vi "Histogram by Bins.vi"(2 "Bins":T1(array[cluster]) {"upper" format="%0.2f"; "lower" format="%0.2f"}, 3 "Input Data":dbl[](array[numeric]) format="%0.2f") -> (0 "# outside":cluster{"total":i32, "above":i32, "below":i32}, 1 "Histogram":i32[](array[numeric]))   [LabVIEW 2020, in "NI_PtbyPt.lvlib"]
uses:
  <vilib>/ptbypt/NI_PtbyPt.lvlib
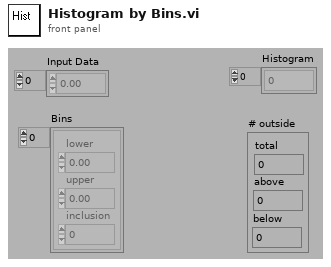
[diagram p1: front panel]
types:
  T1 = cluster{"lower":dbl, "upper":dbl, "inclusion":u32}[]
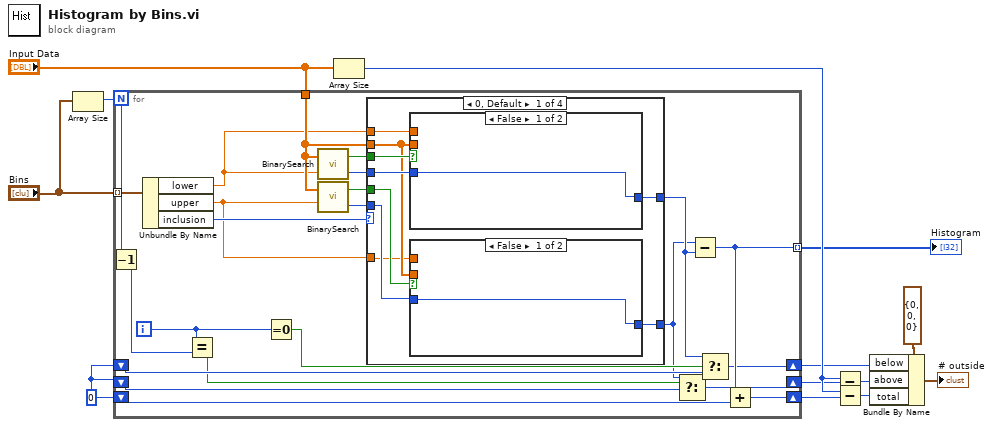
[diagram p0: block diagram]
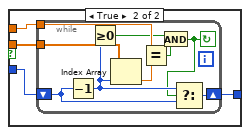
[diagram p2: hidden frame]
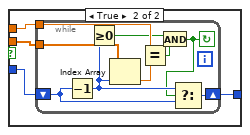
[diagram p3: hidden frame]
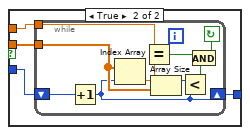
[diagram p5: hidden frame]
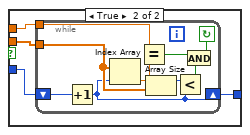
[diagram p6: hidden frame]
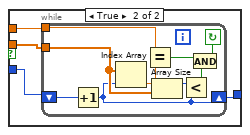
[diagram p8: hidden frame]
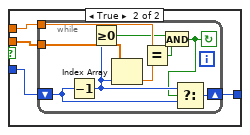
[diagram p9: hidden frame]
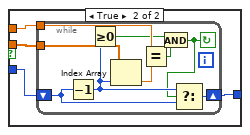
[diagram p11: hidden frame]
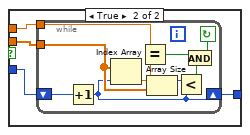
[diagram p12: hidden frame]
diagram:
  w4 = 0
  n1 = Array Size(array="Bins") -> (size(s)=w11:i32)
  n2 = for {
    N: w11 -> [w21]
    tunnel: "Bins" -> [w36] mode=indexing
    tunnel: "Input Data" -> [w31]
    tunnel: [w27] -> w3 mode=indexing
    shift-right: [w28] -> w9
    shift-left: w4 -> [w26]
    shift-right: [w23] -> w7
    shift-left: w4 -> [w24]
    shift-right: [w14] -> w5
    shift-left: w4 -> [w18]
    i -> [w22]
    n3 = Decrement(x=w21) -> (x-1=w20:i32)
    n4 = Unbundle By Name(w36) -> ("lower"=w30:dbl, "upper"=w29:dbl, "inclusion"=w35:u32)
    n5 = Equal?(x=w22, y=w20) -> (x = y?=w19:bool)
    n6 = Equal To 0?(x=w22) -> (x = 0?=w25:bool)
    n7 = call <vilib>:"BinarySearch.vi"("value searching for"=w30, "Sorted Array"=w31) -> ("index"=w17:i32, "isFound"=w32:bool)
    n8 = call <vilib>:"BinarySearch.vi"("value searching for"=w29, "Sorted Array"=w31) -> ("index"=w34:i32, "isFound"=w33:bool)
    n9 = case shown="0, Default" w35 {
      tunnel: w17 -> [w44 w81 w118 w155]
      tunnel: w34 -> [w41 w78 w115 w152]
      tunnel: w33 -> [w43 w80 w117 w154]
      tunnel: w32 -> [w45 w82 w119 w156]
      tunnel: w31 -> [w42 w79 w116 w153]
      tunnel: w30 -> [w40 w77 w114 w151]
      tunnel: w29 -> [w39 w76 w113 w150]
      tunnel: [w38 w75 w112 w149] -> w16
      tunnel: [w37 w74 w111 w148] -> w15
      frame 0, Default {
        n10 = case shown="False" w45 {
          tunnel: w44 -> [w60 w63]
          tunnel: w42 -> [_ w64]
          tunnel: w40 -> [_ w62]
          tunnel: [w60 w61] -> w38
          frame False {
          }
          frame True {
            n11 = while {
              tunnel: w62 -> [w72]
              shift-left: w63 -> [w69]
              shift-right: [w70] -> w61
              tunnel: w64 -> [w73]
              stop <- w65 continue-if-true
              n12 = Decrement(x=w69) -> (x-1=w68:i32)
              n13 = Greater Or Equal To 0?(x=w68) -> (x >= 0?=w67:bool)
              n14 = Index Array(array=w73, index=w68) -> (element=w71:dbl)
              n15 = Equal?(x=w72, y=w71) -> (x = y?=w66:bool)
              n16 = And(x=w67, y=w66) -> (x .and. y?=w65:bool)
              n17 = Select(t=w68, s=w65, f=w69) -> (s? t:f=w70:i32)
            }
          }
        }
        n18 = case shown="False" w43 {
          tunnel: w41 -> [w46 w49]
          tunnel: w42 -> [_ w48]
          tunnel: w39 -> [_ w47]
          tunnel: [w46 w50] -> w37
          frame False {
          }
          frame True {
            n19 = while {
              tunnel: w47 -> [w58]
              shift-left: w49 -> [w55]
              shift-right: [w56] -> w50
              tunnel: w48 -> [w59]
              stop <- w51 continue-if-true
              n20 = Decrement(x=w55) -> (x-1=w54:i32)
              n21 = Greater Or Equal To 0?(x=w54) -> (x >= 0?=w53:bool)
              n22 = Index Array(array=w59, index=w54) -> (element=w57:dbl)
              n23 = Equal?(x=w58, y=w57) -> (x = y?=w52:bool)
              n24 = And(x=w53, y=w52) -> (x .and. y?=w51:bool)
              n25 = Select(t=w54, s=w51, f=w55) -> (s? t:f=w56:i32)
            }
          }
        }
      }
      frame 1 {
        n26 = case shown="False" w82 {
          tunnel: w81 -> [w97 w100]
          tunnel: w79 -> [_ w101]
          tunnel: w77 -> [_ w99]
          tunnel: [w97 w98] -> w75
          frame False {
          }
          frame True {
            n27 = while {
              tunnel: w99 -> [w110]
              shift-left: w100 -> [w108]
              shift-right: [w104] -> w98
              tunnel: w101 -> [w105]
              stop <- w107 continue-if-true
              n28 = Increment(x=w108) -> (x+1=w104:i32)
              n29 = Index Array(array=w105, index=w104) -> (element=w109:dbl)
              n30 = Equal?(x=w110, y=w109) -> (x = y?=w106:bool)
              n31 = Array Size(array=w105) -> (size(s)=w103:i32)
              n32 = Less?(x=w103, y=w104) -> (x < y?=w102:bool)
              n33 = And(x=w106, y=w102) -> (x .and. y?=w107:bool)
            }
          }
        }
        n34 = case shown="False" w80 {
          tunnel: w78 -> [w83 w85]
          tunnel: w79 -> [_ w86]
          tunnel: w76 -> [_ w87]
          tunnel: [w83 w84] -> w74
          frame False {
          }
          frame True {
            n35 = while {
              tunnel: w87 -> [w96]
              shift-left: w85 -> [w94]
              shift-right: [w90] -> w84
              tunnel: w86 -> [w91]
              stop <- w93 continue-if-true
              n36 = Increment(x=w94) -> (x+1=w90:i32)
              n37 = Index Array(array=w91, index=w90) -> (element=w95:dbl)
              n38 = Equal?(x=w96, y=w95) -> (x = y?=w92:bool)
              n39 = Array Size(array=w91) -> (size(s)=w89:i32)
              n40 = Less?(x=w89, y=w90) -> (x < y?=w88:bool)
              n41 = And(x=w92, y=w88) -> (x .and. y?=w93:bool)
            }
          }
        }
      }
      frame 2 {
        n42 = case shown="False" w119 {
          tunnel: w118 -> [w134 w136]
          tunnel: w116 -> [_ w137]
          tunnel: w114 -> [_ w138]
          tunnel: [w134 w135] -> w112
          frame False {
          }
          frame True {
            n43 = while {
              tunnel: w138 -> [w146]
              shift-left: w136 -> [w143]
              shift-right: [w144] -> w135
              tunnel: w137 -> [w147]
              stop <- w139 continue-if-true
              n44 = Decrement(x=w143) -> (x-1=w142:i32)
              n45 = Greater Or Equal To 0?(x=w142) -> (x >= 0?=w141:bool)
              n46 = Index Array(array=w147, index=w142) -> (element=w145:dbl)
              n47 = Equal?(x=w146, y=w145) -> (x = y?=w140:bool)
              n48 = And(x=w141, y=w140) -> (x .and. y?=w139:bool)
              n49 = Select(t=w142, s=w139, f=w143) -> (s? t:f=w144:i32)
            }
          }
        }
        n50 = case shown="False" w117 {
          tunnel: w115 -> [w120 w122]
          tunnel: w116 -> [_ w123]
          tunnel: w113 -> [_ w124]
          tunnel: [w120 w121] -> w111
          frame False {
          }
          frame True {
            n51 = while {
              tunnel: w124 -> [w133]
              shift-left: w122 -> [w131]
              shift-right: [w127] -> w121
              tunnel: w123 -> [w128]
              stop <- w130 continue-if-true
              n52 = Increment(x=w131) -> (x+1=w127:i32)
              n53 = Index Array(array=w128, index=w127) -> (element=w132:dbl)
              n54 = Equal?(x=w133, y=w132) -> (x = y?=w129:bool)
              n55 = Array Size(array=w128) -> (size(s)=w126:i32)
              n56 = Less?(x=w126, y=w127) -> (x < y?=w125:bool)
              n57 = And(x=w129, y=w125) -> (x .and. y?=w130:bool)
            }
          }
        }
      }
      frame 3 {
        n58 = case shown="False" w156 {
          tunnel: w155 -> [w171 w173]
          tunnel: w153 -> [_ w174]
          tunnel: w151 -> [_ w175]
          tunnel: [w171 w172] -> w149
          frame False {
          }
          frame True {
            n59 = while {
              tunnel: w175 -> [w184]
              shift-left: w173 -> [w182]
              shift-right: [w178] -> w172
              tunnel: w174 -> [w179]
              stop <- w181 continue-if-true
              n60 = Increment(x=w182) -> (x+1=w178:i32)
              n61 = Index Array(array=w179, index=w178) -> (element=w183:dbl)
              n62 = Equal?(x=w184, y=w183) -> (x = y?=w180:bool)
              n63 = Array Size(array=w179) -> (size(s)=w177:i32)
              n64 = Less?(x=w177, y=w178) -> (x < y?=w176:bool)
              n65 = And(x=w180, y=w176) -> (x .and. y?=w181:bool)
            }
          }
        }
        n66 = case shown="False" w154 {
          tunnel: w152 -> [w157 w160]
          tunnel: w153 -> [_ w159]
          tunnel: w150 -> [_ w158]
          tunnel: [w157 w161] -> w148
          frame False {
          }
          frame True {
            n67 = while {
              tunnel: w158 -> [w169]
              shift-left: w160 -> [w166]
              shift-right: [w167] -> w161
              tunnel: w159 -> [w170]
              stop <- w162 continue-if-true
              n68 = Decrement(x=w166) -> (x-1=w165:i32)
              n69 = Greater Or Equal To 0?(x=w165) -> (x >= 0?=w164:bool)
              n70 = Index Array(array=w170, index=w165) -> (element=w168:dbl)
              n71 = Equal?(x=w169, y=w168) -> (x = y?=w163:bool)
              n72 = And(x=w164, y=w163) -> (x .and. y?=w162:bool)
              n73 = Select(t=w165, s=w162, f=w166) -> (s? t:f=w167:i32)
            }
          }
        }
      }
    }
    n74 = Select(t=w15, s=w19, f=w18) -> (s? t:f=w14:i32)
    n75 = Subtract(x=w15, y=w16) -> (x-y=w27:i32)
    n76 = Select(t=w16, s=w25, f=w24) -> (s? t:f=w23:i32)
    n77 = Add(x=w27, y=w26) -> (x+y=w28:i32)
  }
  "Histogram" <- w3
  n78 = Array Size(array="Input Data") -> (size(s)=w12:i32)
  n79 = Subtract(x=w12, y=w5) -> (x-y=w8:i32)
  n80 = Subtract(x=w12, y=w9) -> (x-y=w10:i32)
  n81 = Bundle By Name(cluster=cluster{"total":i32, "above":i32, "below":i32} {"total"=0, "above"=0, "below"=0} ("# outside"), "below"=w7, "above"=w8, "total"=w10) -> (→"# outside":cluster{"total":i32, "above":i32, "below":i32})
